vi "configure.vi"(8 "error in (no error)":errorcluster, 11 "GenericPlugin in":refnum<class "FPGAWrapperRK110512Fiber_Spiral.lvclass">) -> (0 "error out":errorcluster, 3 "GenericPlugin out":refnum<class "FPGAWrapperRK110512Fiber_Spiral.lvclass">)   [LabVIEW 2010, in "FPGAWrapperRK110512Fiber_Spiral.lvclass"]
doc: "The dynamic dispatch version of this VI loads and displays the configuration file associated with the plug-in object. The user modify and save the configuration data."
uses:
  FPGAWrapperRK110512Fiber_Spiral.lvclass
  FPGAWrapperRK110512Fiber_Spiral.lvclass/FPGAWrapperRK110512Fiber_Spiral.ctl
  common/classes/GenericComponent/GenericComponent/GenericComponent.lvclass
panel:
  in  "FPGA clock":u32
  in  "Enable ADC clock":bool=TRUE
  in  "cancelButton":bool
  in  "okButton":bool
  out "configuration":string
  in  "ADC clock phase":u8 max=2
  in  "HIFO ADC version":i16=2 min=1 max=2
  # "Configure FPGAWrapperRK120511Fiber_Spiral"
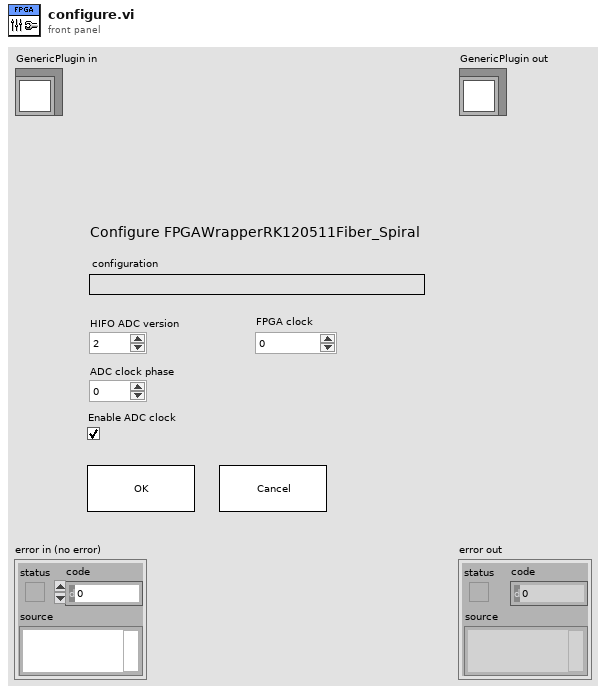
[diagram p1: front panel]
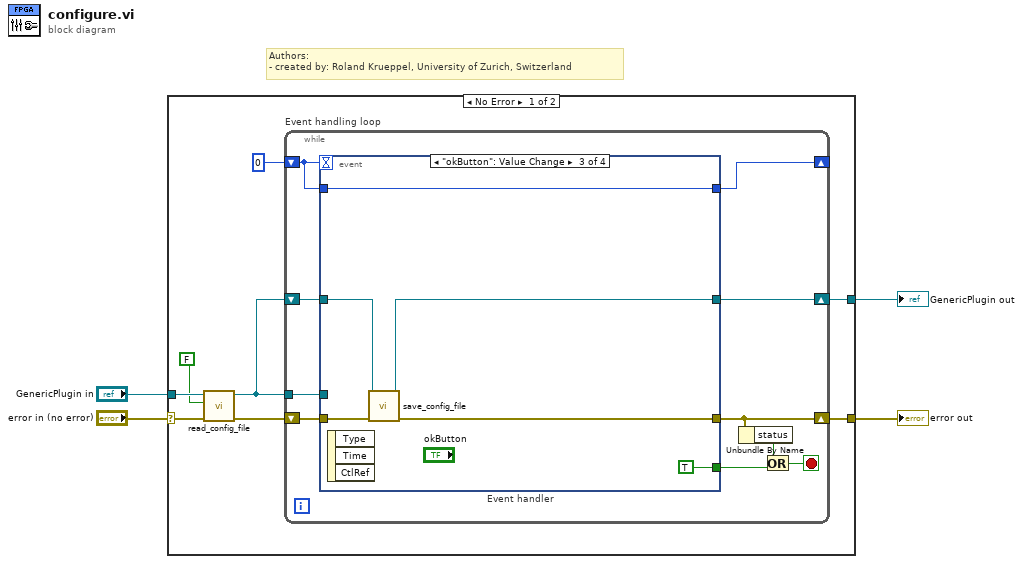
[diagram p0: block diagram]
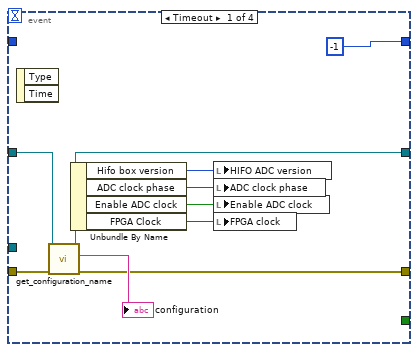
[diagram p2: hidden frame]
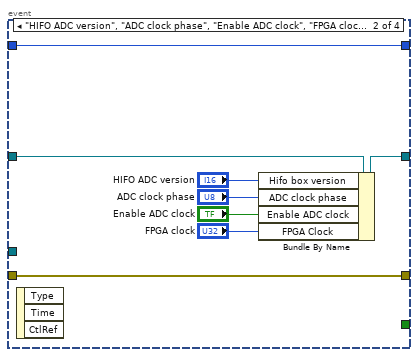
[diagram p3: hidden frame]
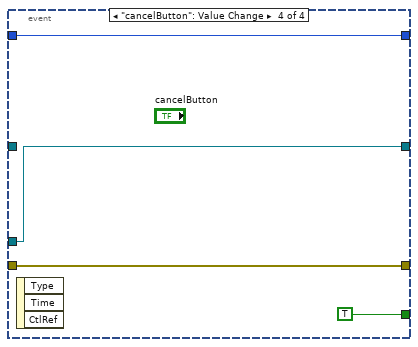
[diagram p4: hidden frame]
diagram:
  # "Authors: \n- created by: Roland Krueppel, University of Zurich, Switzerland"
  n1 = case shown="No Error" "error in (no error)" {
    selector: "error in (no error)" -> [w12 w52]
    tunnel: "GenericPlugin in" -> [w11 w51]
    tunnel: [w7 w51] -> w2
    tunnel: [w6 w52] -> w1
    frame No Error {
      n2 = call-dynamic "read_config_file.vi"("error in (no error)"=w12, "force load?"=FALSE, "GenericPlugin in"=w11) -> ("error out"=w9:errorcluster, "GenericPlugin out"=w8:refnum<class "FPGAWrapperRK110512Fiber_Spiral.lvclass">)  [unwired: 7 in]
      n3 = while "Event handling loop" {
        tunnel: w8 -> [w21]
        shift-right: [w16] -> w6
        shift-left: w9 -> [w22]
        shift-right: [w19] -> w7
        shift-left: w8 -> [w20]
        shift-right: [w17] -> _
        shift-left: 0 -> [w18]
        stop <- w13 stop-if-true
        n4 = event "Event handler" shown="[2] \"okButton\": Value Change" {
          selector: _ -> [_ _ _ _]
          dyn-events: _ -> [_ _ _ _]
          timeout: w18 -> [_ _ _ _]
          tunnel: w22 -> [w32 w40 w46 w49]
          tunnel: w21 -> [_ _ _ w50]
          tunnel: w20 -> [w30 w39 w45 _]
          tunnel: [w29 w38 w43 w50] -> w19
          tunnel: w18 -> [_ w34 w42 w48]
          tunnel: [-1 w34 w42 w48] -> w17
          tunnel: [w24 w40 w44 w49] -> w16
          tunnel: [_ _ TRUE ("y") TRUE ("y")] -> w14
          event Timeout {
            n5 = event-data() -> ()  [unwired: 1 in, 2 out]
            n6 = call "get_configuration_name.vi"("error in (no error)"=w32, "GenericPlugin.lvclass in"=w30) -> ("error out"=w24:errorcluster, "configuration name"=→"configuration":string, "GenericPlugin.lvclass out"=w29:refnum<class "FPGAWrapperRK110512Fiber_Spiral.lvclass">)  [unwired: 7 in]
            n7 = Unbundle By Name(w29) -> ("Hifo box version"=w28:i16, "ADC clock phase"=w27:u8, "Enable ADC clock"=w26:bool, "FPGA Clock"=w23:u32)
            n8 = local write "HIFO ADC version"(w28) -> ()
            n9 = local write "ADC clock phase"(w27) -> ()
            n10 = local write "Enable ADC clock"(w26) -> ()
            n11 = local write "FPGA clock"(w23) -> ()
          }
          event "HIFO ADC version", "ADC clock phase", "Enable ADC clock", "FPGA clock": Value Change {
            n12 = event-data() -> ()  [unwired: 1 in, 3 out]
            n13 = Bundle By Name(cluster=w39, "Hifo box version"="HIFO ADC version", "ADC clock phase"="ADC clock phase", "Enable ADC clock"="Enable ADC clock", "FPGA Clock"="FPGA clock") -> (w38:refnum<class "FPGAWrapperRK110512Fiber_Spiral.lvclass">)
          }
          event "okButton": Value Change {
            n14 = event-data() -> ()  [unwired: 1 in, 3 out]
            n15 = call-dynamic "save_config_file.vi"("error in (no error)"=w46, "GenericPlugin in"=w45) -> ("error out"=w44:errorcluster, "GenericPlugin out"=w43:refnum<class "FPGAWrapperRK110512Fiber_Spiral.lvclass">)  [unwired: 8 in]
          }
          event "cancelButton": Value Change {
            n16 = event-data() -> ()  [unwired: 1 in, 3 out]
          }
        }
        n17 = Unbundle By Name(w16) -> ("status"=w15:bool)
        n18 = Or(x=w15, y=w14) -> (x .or. y?=w13:bool)
      }
    }
    frame Error {
    }
  }
  "error out" <- w1
  "GenericPlugin out" <- w2
